vi "Vision Research Phantom Series PhFile PhPrintTime.vi"(0 "CH [in]":u64, 1 "ImNo":i32, 2 "Options":u32(ring) items=["PPT_UT"=1, "PPT_UT_DATE"=2, "PPT_UT_TIME"=3, "PPT_UT_FRAC"=4, "PPT_UT_ATTRIB"=5, "PPT_LT"=10, "PPT_LT_DATE"=11, "PPT_LT_TIME"=12, "PPT_LT_FRAC"=13, "PPT_LT_ATTRIB"=14, "PPT_SMPTETC"=20], 5 "Error In (no error)":errorcluster) -> (16 "szTime":path, 19 "Error Out":errorcluster)   [LabVIEW 2013, in "VRI.lvlib"]
doc: "PhPrintTime\nHRESULT PhPrintTime(CINEHANDLE hC, INT ImNo, UINT Options, PSTR szTime);\n\nParameters\nCH [in]\n The cine for which time information is requested.\nImNo [in]\n The cine image number the time is requested for.\nOptions [in, optional]\n Numerical value specifying time format options. \nszTime [out]\n Char buffer to be filled with time data according to the specified format.\n\nReturn Value\nThe function returns ERR_Ok in case of success or an error code, otherwise. To get extended error information call PhGetErrorMessage.\n\nRemarks\nPrints the time for the given cine image according to current cine time format and specified format options. To control the time format, use PhSetCineInfo/PhGetCineInfo and the GCI_TIMEFORMAT selector.\nTime format options are supported only for TF_LT and TF_UT time formats. For TF_SMPTE format, the time is always printed in full.\n\nRequired Header\nPhFile.h"
uses:
  VRI.lvlib
  Phantom DLLs/PhFile.dll
panel:
  # "For instructions on the use of this VI, press Ctrl+H to display the help window and move the mouse over the icon, controls, and indicators"
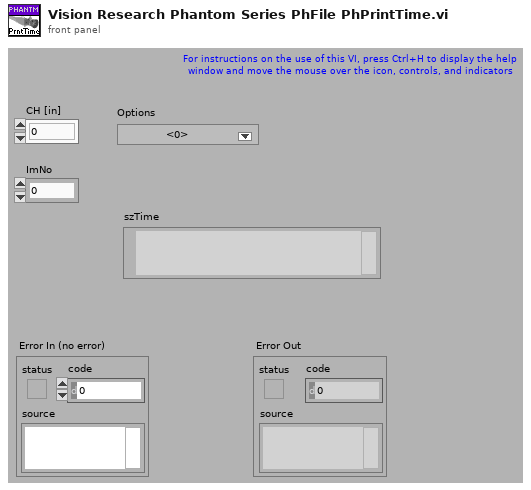
[diagram p1: front panel]
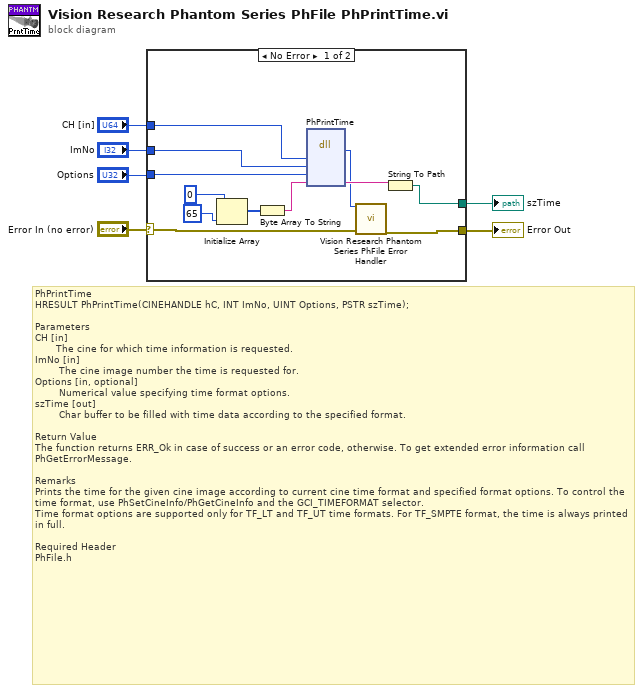
[diagram p0: block diagram]
diagram:
  # "PhPrintTime\nHRESULT PhPrintTime(CINEHANDLE hC, INT ImNo, UINT Options, PSTR szTime);\n\nParameters\nCH [in]\n\t      The cine for which time information is requested.\nImNo [in]\n\t\t      The cine image number the time is requested for.\nOptions [in, optional]\n\t       Numerical value specifying time format options. \nszTime [out]\n\t       Char buffer to be filled with time data according to the specified format.\n\nReturn Value\nThe function returns ERR_Ok in case of success or an error code, otherwise. To get extended error information call PhGetErrorMessage.\n\nRemarks\nPrints the time for the given cine image according to current cine time format and specified format options. To control the time format, use PhSetCineInfo/PhGetCineInfo and the GCI_TIMEFORMAT selector.\nTime format options are supported only for TF_LT and TF_UT time formats. For TF_SMPTE format, the time is always printed in full.\n\nRequired Header\nPhFile.h"
  n1 = case shown="No Error" "Error In (no error)" {
    selector: "Error In (no error)" -> [w18 w19]
    tunnel: [w17 w19] -> w5
    tunnel: [w16 _] -> w3
    tunnel: "Options" -> [w15 _]
    tunnel: "ImNo" -> [w14 _]
    tunnel: "CH [in]" -> [w13 _]
    frame No Error {
      n2 = Initialize Array(u8 0, 65 ("dimension size")) -> (w11:u8[])
      n3 = Byte Array To String(unsigned byte array=w11) -> (string=w9:string)
      n4 = dll-call lib="C:/Projects/SDK/32-bit/Vision Research Phantom Series Labview Driver/Phantom DLLs/PhFile.dll" fn="PhPrintTime"("hC"=w13, "ImNo"=w14, "Options"=w15, "szTime"=w9) -> ("return type"=w7:i32, "szTime"=w12:string)  [unwired: 6 in, 2 out]
      n5 = call "Vision Research Phantom Series PhFile Error Handler.vi"("Error Code (0)"=w7, "Error In (no error)"=w18) -> ("Error Out"=w17:errorcluster)  [unwired: 17 out]
      n6 = String To Path(string=w12) -> (path=w16:path)
    }
    frame Error {
    }
  }
  "Error Out" <- w5
  "szTime" <- w3
